vi "API - Set Rx Packet Properties.vi"(8 "error in (no error)":errorcluster, 10 "Rx Packet Info":T1 {"Channels"."Destination Ref" format="%.0x"}, 11 "Packet Ref In":T3=18446744073709551615 format="%.0x") -> (0 "error out":errorcluster, 3 "Packet Ref Out":T3=18446744073709551615 format="%.0x")   [LabVIEW 2016, in "UDP-Custom-Device System Explorer.lvlib"]
uses:
  UDP-Custom-Device System Explorer.lvlib
  <vilib>/NI Veristand/Custom Device API/Custom Device Item Ref.ctl
  Types/TypeDef - Rx Packet Data.ctl
  TypeDef - Channel Data.ctl
  Shared/DataTypes.ctl
  Shared/Constants.vi
  <vilib>/NI Veristand/Custom Device API/Set Item Property (String Array).vi
  <vilib>/NI Veristand/Custom Device API/Set Item Property (I32).vi
  <vilib>/NI Veristand/Custom Device API/Set Item Property (String).vi
  Shared/UDP-Custom-Device Shared.lvlib
  <vilib>/NI VeriStand/Custom Device API/Custom Device API.lvlib
  <vilib>/NI VeriStand/Custom Device Tools/Custom Device Utility Library/Custom Device Utility Library.lvlib
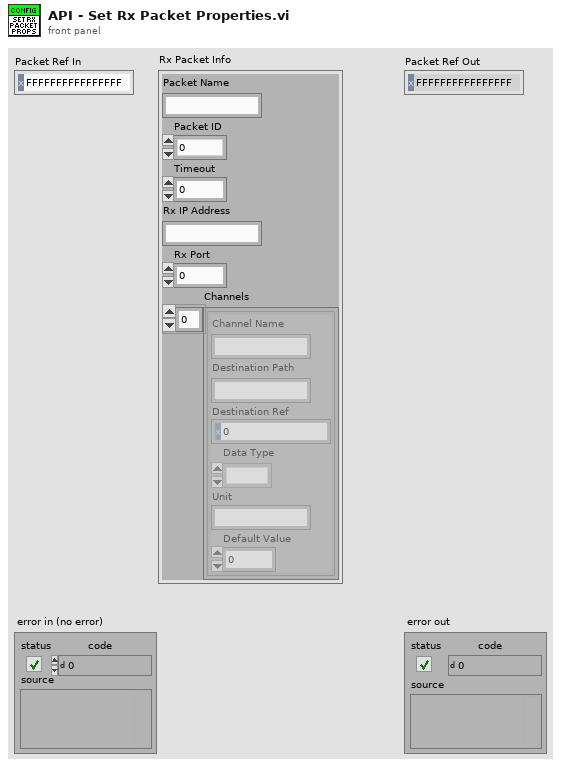
[diagram p1: front panel]
types:
  T1 = typedef "UDP-Custom-Device System Explorer.lvlib/TypeDef - Rx Packet Data.ctl" = cluster{"Packet Name":string, "Packet ID":i32, "Timeout":i32, "Rx IP Address":string, "Rx Port":i32, "Channels":T2[]}
  T2 = typedef "UDP-Custom-Device System Explorer.lvlib/TypeDef - Channel Data.ctl" = cluster{"Channel Name":string, "Destination Path":string, "Destination Ref":T3, "Data Type":T4, "Unit":string, "Default Value":dbl}
  T3 = typedef "Custom Device API.lvlib/Custom Device Item Ref.ctl" = u64
  T4 = typedef "UDP-Custom-Device Shared.lvlib/DataTypes.ctl" = enum16{""}
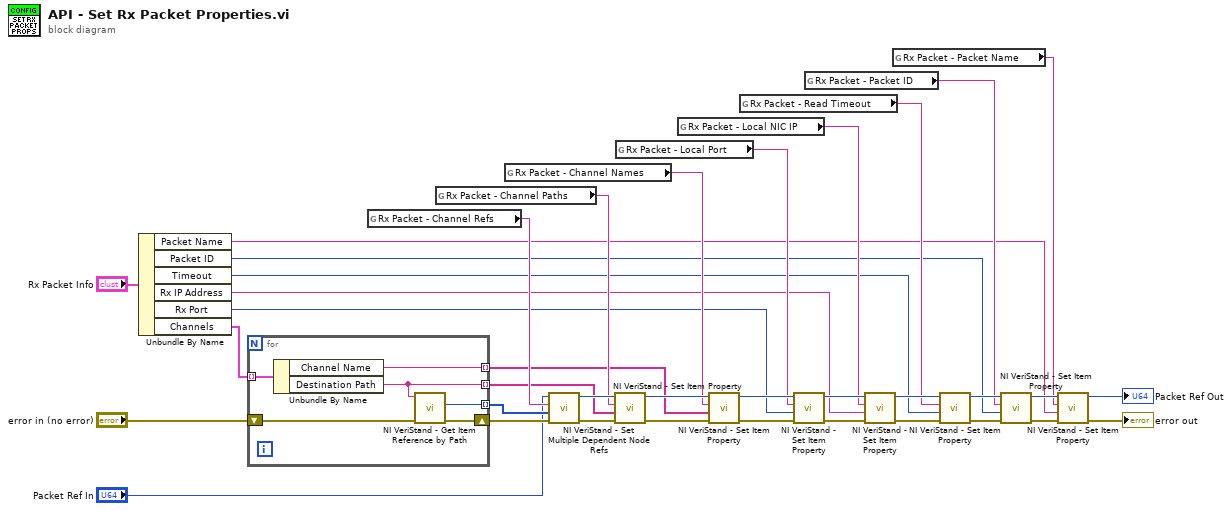
[diagram p0: block diagram]
diagram:
  n1 = Unbundle By Name("Rx Packet Info") -> ("Packet Name"=w6:string, "Packet ID"=w8:i32, "Timeout"=w14:i32, "Rx IP Address"=w16:string, "Rx Port"=w18:i32, "Channels"=w1:T2[])
  n2 = for {
    tunnel: w1 -> [w43] mode=indexing
    tunnel: [w40] -> w22 mode=indexing
    tunnel: [w41] -> w21 mode=indexing
    tunnel: [w39] -> w26 mode=indexing
    shift-right: [w38] -> w36
    shift-left: "error in (no error)" -> [w42]
    n3 = Unbundle By Name(w43) -> ("Channel Name"=w41:string, "Destination Path"=w40:string)
    n4 = call <vilib>:"NI VeriStand - Get Item Reference by Path.vi"("error in (no error)"=w42, "Item Path in"=w40) -> ("error out"=w38:errorcluster, "Item Ref"=w39:T3)  [unwired: 6 in, 2 out]
  }
  n5 = global read "Constants.vi" "Rx Packet - Channel Refs"() -> (w25:string)
  n6 = global read "Constants.vi" "Rx Packet - Channel Paths"() -> (w23:string)
  n7 = global read "Constants.vi" "Rx Packet - Channel Names"() -> (w20:string)
  n8 = call <vilib>:"NI VeriStand - Set Multiple Dependent Node Refs.vi"("error in (no error)"=w36, "Dependent Node Refs"=w26, "Base Property Name"=w25, "Item Ref in"="Packet Ref In") -> ("error out"=w27:errorcluster, "Item Ref out"=w24:T3)  [unwired: 6 in]
  n9 = call-poly <vilib>:"NI VeriStand - Set Item Property.vi"("error in (no error)"=w27, "Value"=w22, "Property Name"=w23, "Item Ref in"=w24) -> ("error out"=w28:errorcluster, "Item Ref out"=w35:T3)  [unwired: 5 in, 1 out]
  n10 = global read "Constants.vi" "Rx Packet - Local Port"() -> (w19:string)
  n11 = global read "Constants.vi" "Rx Packet - Local NIC IP"() -> (w17:string)
  n12 = call-poly <vilib>:"NI VeriStand - Set Item Property.vi"("error in (no error)"=w28, "Value"=w21, "Property Name"=w20, "Item Ref in"=w35) -> ("error out"=w29:errorcluster, "Item Ref out"=w34:T3)  [unwired: 5 in, 1 out]
  n13 = global read "Constants.vi" "Rx Packet - Read Timeout"() -> (w15:string)
  n14 = call-poly <vilib>:"NI VeriStand - Set Item Property.vi"("error in (no error)"=w29, "Value"=w18, "Property Name"=w19, "Item Ref in"=w34) -> ("error out"=w30:errorcluster, "Item Ref out"=w33:T3)  [unwired: 5 in, 1 out]
  n15 = global read "Constants.vi" "Rx Packet - Packet ID"() -> (w9:string)
  n16 = call-poly <vilib>:"NI VeriStand - Set Item Property.vi"("error in (no error)"=w30, "Value"=w16, "Property Name"=w17, "Item Ref in"=w33) -> ("error out"=w31:errorcluster, "Item Ref out"=w32:T3)  [unwired: 5 in, 1 out]
  n17 = global read "Constants.vi" "Rx Packet - Packet Name"() -> (w7:string)
  n18 = call-poly <vilib>:"NI VeriStand - Set Item Property.vi"("error in (no error)"=w31, "Value"=w14, "Property Name"=w15, "Item Ref in"=w32) -> ("error out"=w13:errorcluster, "Item Ref out"=w12:T3)  [unwired: 5 in, 1 out]
  n19 = call-poly <vilib>:"NI VeriStand - Set Item Property.vi"("error in (no error)"=w13, "Value"=w8, "Property Name"=w9, "Item Ref in"=w12) -> ("error out"=w11:errorcluster, "Item Ref out"=w10:T3)  [unwired: 5 in, 1 out]
  n20 = call-poly <vilib>:"NI VeriStand - Set Item Property.vi"("error in (no error)"=w11, "Value"=w6, "Property Name"=w7, "Item Ref in"=w10) -> ("error out"=→"error out":errorcluster, "Item Ref out"=→"Packet Ref Out":T3)  [unwired: 5 in, 1 out]
